vi "Lesson 3 - Exercise 3.1.2 - Freq Orthogonality.vi"() -> ()   [LabVIEW 2015]
uses:
  <vilib>/Analysis/NI_AALBase.lvlib
panel:
  in  "B":dbl=2.0
  in  "B Deg":dbl min=-360.0 max=360.0 step=5.0
  out "Sin(A) & Sin(B)":dbl[][](graph)=[[0.0, 0.12533323356430426, 0.24868988716485482, 0.368124552684678, 0.4817536741017153, 0.5877852522924731, 0.6845471059286887, 0.7705132427757893, 0.8443279255020152, 0.9048270524660196, 0.9510565162951536, 0.9822872507286887, 0.9980267284282716, 0.9980267284282716, 0.9822872507286886, 0.9510565162951535, 0.9048270524660195, 0.844327925502015, 0.7705132427757891, 0.6845471059286885, 0.587785252292473, 0.48175367410171505, 0.3681245526846778, 0.24868988716485452, 0.12533323356430404, -3.055146196792591e-16, -0.1253332335643045, -0.2486898871648551, -0.36812455268467825, -0.4817536741017156, -0.5877852522924735, -0.684547105928689, -0.7705132427757896, -0.8443279255020153, -0.9048270524660198, -0.9510565162951538, -0.9822872507286888, -0.9980267284282717, -0.9980267284282716, -0.9822872507286886, -0.9510565162951534, -0.9048270524660194, -0.8443279255020149, -0.7705132427757889, -0.6845471059286883, -0.5877852522924727, -0.48175367410171477, -0.3681245526846774, -0.2486898871648542, -0.12533323356430362, 6.254084706711072e-16, 0.12533323356430492, 0.24868988716485543, 0.36812455268467864, 0.4817536741017159, 0.5877852522924738, 0.6845471059286892, 0.7705132427757898, 0.8443279255020154, 0.9048270524660199, 0.9510565162951538, 0.9822872507286888, 0.9980267284282716, 0.9980267284282716, 0.9822872507286885, 0.9510565162951533, 0.9048270524660191, 0.8443279255020146, 0.7705132427757887, 0.6845471059286881, 0.5877852522924725, 0.4817536741017145, 0.3681245526846772, 0.24868988716485388, 0.1253332335643034, -9.78736406156977e-16, -0.12533323356430512, -0.24868988716485577, -0.3681245526846788, -0.4817536741017162, -0.5877852522924739, -0.6845471059286895, -0.7705132427757899, -0.8443279255020157, -0.90482705246602, -0.951056516295154, -0.9822872507286889, -0.9980267284282717, -0.9980267284282716, -0.9822872507286885, -0.9510565162951533, -0.904827052466019, -0.8443279255020145, -0.7705132427757885, -0.6845471059286878, -0.5877852522924721, -0.4817536741017142, -0.3681245526846768, -0.24868988716485357, -0.12533323356430298], [0.0, 0.12533323356430426, 0.24868988716485482, 0.368124552684678, 0.4817536741017153, 0.5877852522924731, 0.6845471059286887, 0.7705132427757893, 0.8443279255020152, 0.9048270524660196, 0.9510565162951536, 0.9822872507286887, 0.9980267284282716, 0.9980267284282716, 0.9822872507286886, 0.9510565162951535, 0.9048270524660195, 0.844327925502015, 0.7705132427757891, 0.6845471059286885, 0.587785252292473, 0.48175367410171505, 0.3681245526846778, 0.24868988716485452, 0.12533323356430404, -3.055146196792591e-16, -0.1253332335643045, -0.2486898871648551, -0.36812455268467825, -0.4817536741017156, -0.5877852522924735, -0.684547105928689, -0.7705132427757896, -0.8443279255020153, -0.9048270524660198, -0.9510565162951538, -0.9822872507286888, -0.9980267284282717, -0.9980267284282716, -0.9822872507286886, -0.9510565162951534, -0.9048270524660194, -0.8443279255020149, -0.7705132427757889, -0.6845471059286883, -0.5877852522924727, -0.48175367410171477, -0.3681245526846774, -0.2486898871648542, -0.12533323356430362, 6.254084706711072e-16, 0.12533323356430492, 0.24868988716485543, 0.36812455268467864, 0.4817536741017159, 0.5877852522924738, 0.6845471059286892, 0.7705132427757898, 0.8443279255020154, 0.9048270524660199, 0.9510565162951538, 0.9822872507286888, 0.9980267284282716, 0.9980267284282716, 0.9822872507286885, 0.9510565162951533, 0.9048270524660191, 0.8443279255020146, 0.7705132427757887, 0.6845471059286881, 0.5877852522924725, 0.4817536741017145, 0.3681245526846772, 0.24868988716485388, 0.1253332335643034, -9.78736406156977e-16, -0.12533323356430512, -0.24868988716485577, -0.3681245526846788, -0.4817536741017162, -0.5877852522924739, -0.6845471059286895, -0.7705132427757899, -0.8443279255020157, -0.90482705246602, -0.951056516295154, -0.9822872507286889, -0.9980267284282717, -0.9980267284282716, -0.9822872507286885, -0.9510565162951533, -0.904827052466019, -0.8443279255020145, -0.7705132427757885, -0.6845471059286878, -0.5877852522924721, -0.4817536741017142, -0.3681245526846768, -0.24868988716485357, -0.12533323356430298]]
  in  "A":dbl=2.0
  in  "stop":bool
  out "SUM[SinA (*) SinB+deg]":dbl=8.743006318923108e-16 format="%.2f"
  out "Sin(A) * Sin(B)":dbl[][](graph)
  out "Sin(B)":dbl[](graph)=[0.0, 0.12533323356430426, 0.24868988716485482, 0.368124552684678, 0.4817536741017153, 0.5877852522924731, 0.6845471059286887, 0.7705132427757893, 0.8443279255020152, 0.9048270524660196, 0.9510565162951536, 0.9822872507286887, 0.9980267284282716, 0.9980267284282716, 0.9822872507286886, 0.9510565162951535, 0.9048270524660195, 0.844327925502015, 0.7705132427757891, 0.6845471059286885, 0.587785252292473, 0.48175367410171505, 0.3681245526846778, 0.24868988716485452, 0.12533323356430404, -3.055146196792591e-16, -0.1253332335643045, -0.2486898871648551, -0.36812455268467825, -0.4817536741017156, -0.5877852522924735, -0.684547105928689, -0.7705132427757896, -0.8443279255020153, -0.9048270524660198, -0.9510565162951538, -0.9822872507286888, -0.9980267284282717, -0.9980267284282716, -0.9822872507286886, -0.9510565162951534, -0.9048270524660194, -0.8443279255020149, -0.7705132427757889, -0.6845471059286883, -0.5877852522924727, -0.48175367410171477, -0.3681245526846774, -0.2486898871648542, -0.12533323356430362, 6.254084706711072e-16, 0.12533323356430492, 0.24868988716485543, 0.36812455268467864, 0.4817536741017159, 0.5877852522924738, 0.6845471059286892, 0.7705132427757898, 0.8443279255020154, 0.9048270524660199, 0.9510565162951538, 0.9822872507286888, 0.9980267284282716, 0.9980267284282716, 0.9822872507286885, 0.9510565162951533, 0.9048270524660191, 0.8443279255020146, 0.7705132427757887, 0.6845471059286881, 0.5877852522924725, 0.4817536741017145, 0.3681245526846772, 0.24868988716485388, 0.1253332335643034, -9.78736406156977e-16, -0.12533323356430512, -0.24868988716485577, -0.3681245526846788, -0.4817536741017162, -0.5877852522924739, -0.6845471059286895, -0.7705132427757899, -0.8443279255020157, -0.90482705246602, -0.951056516295154, -0.9822872507286889, -0.9980267284282717, -0.9980267284282716, -0.9822872507286885, -0.9510565162951533, -0.904827052466019, -0.8443279255020145, -0.7705132427757885, -0.6845471059286878, -0.5877852522924721, -0.4817536741017142, -0.3681245526846768, -0.24868988716485357, -0.12533323356430298]
  out "Sin(A)":dbl[](graph)=[0.0, 0.12533323356430426, 0.24868988716485482, 0.368124552684678, 0.4817536741017153, 0.5877852522924731, 0.6845471059286887, 0.7705132427757893, 0.8443279255020152, 0.9048270524660196, 0.9510565162951536, 0.9822872507286887, 0.9980267284282716, 0.9980267284282716, 0.9822872507286886, 0.9510565162951535, 0.9048270524660195, 0.844327925502015, 0.7705132427757891, 0.6845471059286885, 0.587785252292473, 0.48175367410171505, 0.3681245526846778, 0.24868988716485452, 0.12533323356430404, -3.055146196792591e-16, -0.1253332335643045, -0.2486898871648551, -0.36812455268467825, -0.4817536741017156, -0.5877852522924735, -0.684547105928689, -0.7705132427757896, -0.8443279255020153, -0.9048270524660198, -0.9510565162951538, -0.9822872507286888, -0.9980267284282717, -0.9980267284282716, -0.9822872507286886, -0.9510565162951534, -0.9048270524660194, -0.8443279255020149, -0.7705132427757889, -0.6845471059286883, -0.5877852522924727, -0.48175367410171477, -0.3681245526846774, -0.2486898871648542, -0.12533323356430362, 6.254084706711072e-16, 0.12533323356430492, 0.24868988716485543, 0.36812455268467864, 0.4817536741017159, 0.5877852522924738, 0.6845471059286892, 0.7705132427757898, 0.8443279255020154, 0.9048270524660199, 0.9510565162951538, 0.9822872507286888, 0.9980267284282716, 0.9980267284282716, 0.9822872507286885, 0.9510565162951533, 0.9048270524660191, 0.8443279255020146, 0.7705132427757887, 0.6845471059286881, 0.5877852522924725, 0.4817536741017145, 0.3681245526846772, 0.24868988716485388, 0.1253332335643034, -9.78736406156977e-16, -0.12533323356430512, -0.24868988716485577, -0.3681245526846788, -0.4817536741017162, -0.5877852522924739, -0.6845471059286895, -0.7705132427757899, -0.8443279255020157, -0.90482705246602, -0.951056516295154, -0.9822872507286889, -0.9980267284282717, -0.9980267284282716, -0.9822872507286885, -0.9510565162951533, -0.904827052466019, -0.8443279255020145, -0.7705132427757885, -0.6845471059286878, -0.5877852522924721, -0.4817536741017142, -0.3681245526846768, -0.24868988716485357, -0.12533323356430298]
  # "*Set A or B to any value\n   -Observe the cancelation\n   -Results in a summation to zero"
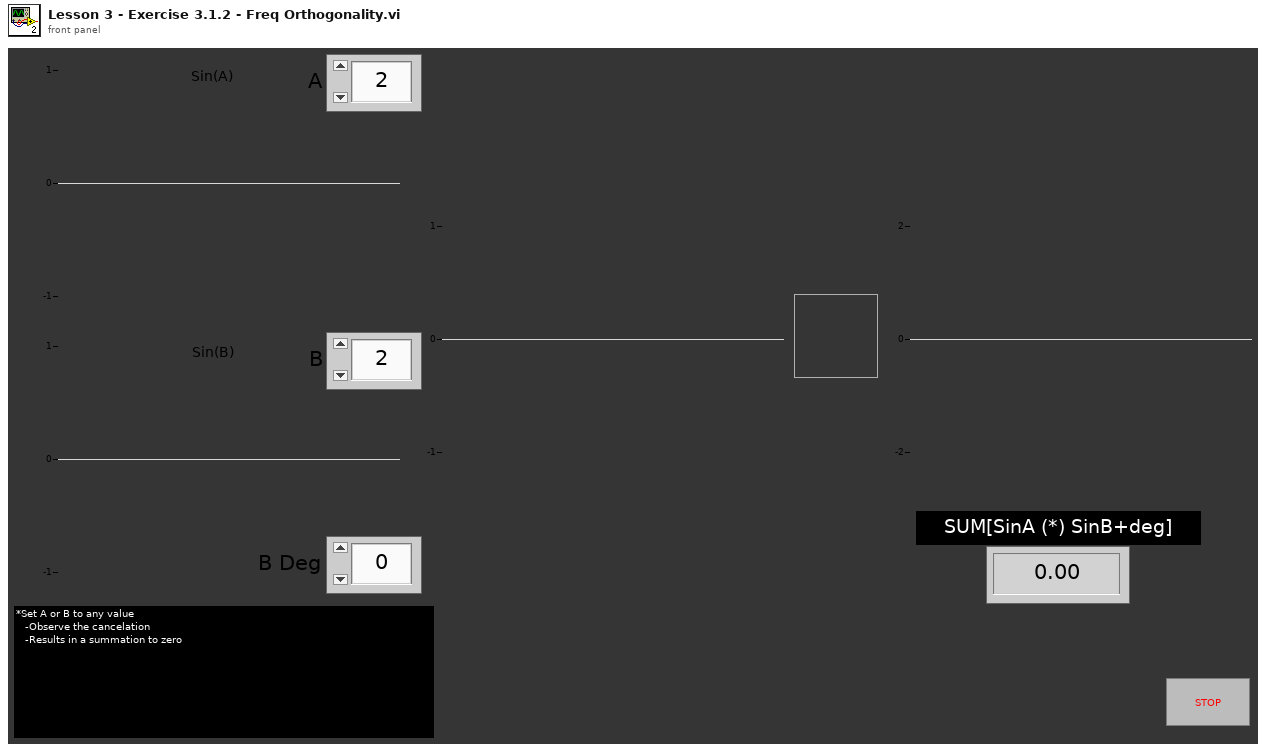
[diagram p1: front panel]
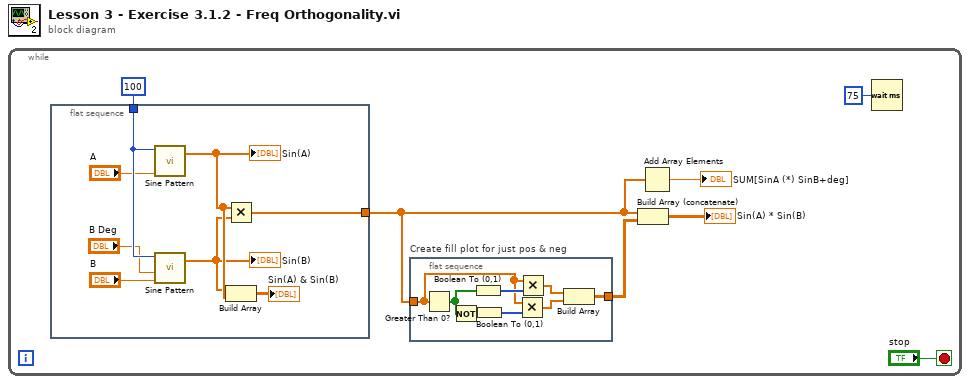
[diagram p0: block diagram]
diagram:
  n1 = while {
    stop <- "stop" stop-if-true
    n2 = flat-sequence {
      tunnel: [w23] -> w1
      tunnel: 100 ("samples") -> [w22]
      frame #0 {
        n3 = call <vilib>:"Sine Pattern.vi"("cycles"="A", "samples"=w22) -> ("Sinusoidal Pattern"=w18:dbl[])  [unwired: 2 in, 1 out]
        "Sin(A)" <- w18
        n4 = call <vilib>:"Sine Pattern.vi"("cycles"="B", "phase(degrees)"="B Deg", "samples"=w22) -> ("Sinusoidal Pattern"=w17:dbl[])  [unwired: 1 in, 1 out]
        "Sin(B)" <- w17
        n5 = Multiply(x=w18, y=w17) -> (x*y=w23:dbl[])
        n6 = Build Array(w17, w18) -> (→"Sin(A) & Sin(B)":dbl[][])
      }
    }
    n7 = flat-sequence "Create fill plot for just pos & neg" {
      tunnel: w1 -> [w8]
      tunnel: [w9] -> w2
      frame #0 {
        n8 = Greater Than 0?(x=w8) -> (x > 0?=w13:bool[])
        n9 = Not(x=w13) -> (.not. x?=w12:bool[])
        n10 = Boolean To (0,1)(Boolean=w13) -> (0, 1=w15:i16[])
        n11 = Boolean To (0,1)(Boolean=w12) -> (0, 1=w11:i16[])
        n12 = Multiply(x=w8, y=w11) -> (x*y=w10:dbl[])
        n13 = Multiply(x=w8, y=w15) -> (x*y=w14:dbl[])
        n14 = Build Array(w14, w10) -> (w9:dbl[][])
      }
    }
    n15 = Build Array (concatenate)(w1, w2) -> (→"Sin(A) * Sin(B)":dbl[][])
    n16 = Add Array Elements(numeric array=w1) -> (sum=→"SUM[SinA (*) SinB+deg]":dbl)
    n17 = Wait (ms)(milliseconds to wait=u32 75) -> ()  [unwired: 1 out]
  }
